vi "dfd_Convert ZPK String to Filter.vi"(8 "error in (no error)":errorcluster, 10 "xml string in":string, 11 "filter":T1={"mSRate_Fs"=1.0, "mSRate_Version"="1.0", "mSRate_Comments"="", "mSRate_OrgCoef"={"type"=enum."Undefined", "gain"=1.0, "coef a (k)"=[], "coef b (v)"=[]}, "mSRate_CurCoef"={"type"=enum."Undefined", "gain"=1.0, "coef a (k)"=[], "coef b (v)"=[]}, "mSRate_Quantized?"=FALSE, "mSRate_QCoef"={"type"=enum."Undefined", "gain"=1.0, "coef a (k)"=[], "coef b (v)"=[]}, "mSRate_QSettings"=[], "mSRate_Order"=0, "mSRate_Scaling"={"mSRate_ScaleByPowerOf2?"=FALSE, "mSRate_ScaleType"=enum."No Norm"}} {"mSRate_QSettings"."source" items=["Coef a/k"=0, "Coef b/v"=7, "Input"=1, "Output"=2, "Multiplicand"=3, "Product"=4, "Sum"=5, "Delay"=6, "Gain"=8]}) -> (0 "error out":errorcluster, 3 "filter out":T1={"mSRate_Fs"=1.0, "mSRate_Version"="1.0", "mSRate_Comments"="", "mSRate_OrgCoef"={"type"=enum."Undefined", "gain"=1.0, "coef a (k)"=[], "coef b (v)"=[]}, "mSRate_CurCoef"={"type"=enum."Undefined", "gain"=1.0, "coef a (k)"=[], "coef b (v)"=[]}, "mSRate_Quantized?"=FALSE, "mSRate_QCoef"={"type"=enum."Undefined", "gain"=1.0, "coef a (k)"=[], "coef b (v)"=[]}, "mSRate_QSettings"=[], "mSRate_Order"=0, "mSRate_Scaling"={"mSRate_ScaleByPowerOf2?"=FALSE, "mSRate_ScaleType"=enum."No Norm"}} {"mSRate_QSettings"."source" items=["Coef a/k"=0, "Coef b/v"=7, "Input"=1, "Output"=2, "Multiplicand"=3, "Product"=4, "Sum"=5, "Delay"=6, "Gain"=8]})   [LabVIEW 2017, in "NI_DigFilter_Process.lvlib"]
uses:
  <vilib>/addons/Digital Filter Design/NI_DigFilter_Process.lvlib
  <vilib>/addons/Digital Filter Design/_Objects.llb/DFD Filter Obj.ctl
  <vilib>/addons/Digital Filter Design/_Objects.llb/DFD Filter Coef.ctl
  <vilib>/addons/Digital Filter Design/_Objects.llb/DFD Filter Structure Type Selector.ctl
  <vilib>/addons/Digital Filter Design/_Objects.llb/dfd_Internal Quantization Settings.ctl
  <vilib>/addons/Digital Filter Design/_Objects.llb/dfd_Internal Quantization Srcs.ctl
  <vilib>/addons/Digital Filter Design/_Objects.llb/DFD Coef Norm Type.ctl
  <vilib>/addons/Digital Filter Design/NI_DigFilterLicensed.lvlib
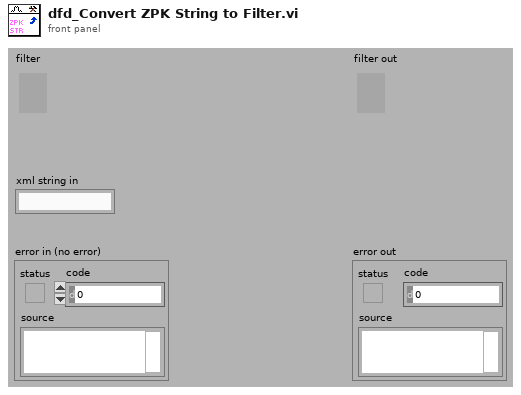
[diagram p1: front panel]
types:
  T1 = typedef "NI_DigFilterLicensed.lvlib/DFD Filter Obj.ctl" = cluster{"mSRate_Fs":dbl, "mSRate_Version":string, "mSRate_Comments":string, "mSRate_OrgCoef":T2, "mSRate_CurCoef":T2, "mSRate_Quantized?":bool, "mSRate_QCoef":T2, "mSRate_QSettings":T4[], "mSRate_Order":i32, "mSRate_Scaling":cluster{"mSRate_ScaleByPowerOf2?":bool, "mSRate_ScaleType":T6}}
  T2 = typedef "NI_DigFilterLicensed.lvlib/DFD Filter Coef.ctl" = cluster{"type":T3, "gain":dbl, "coef a (k)":dbl[], "coef b (v)":dbl[]}
  T3 = typedef "NI_DigFilterLicensed.lvlib/DFD Filter Structure Type Selector.ctl" = enum16{"Undefined", "FIR Direct Form", "FIR Direct Form Transposed", "FIR Symmetric", "FIR Antisymmetric", "IIR Direct Form I", "IIR Direct Form I Transposed", "IIR Direct Form II", "IIR Direct Form II Transposed", "IIR Cascaded Second Order Sections Form I", "IIR Cascaded Second Order Sections Form I Transposed", "IIR Cascaded Second Order Sections Form II", "IIR Cascaded Second Order Sections Form II Transposed", "Lattice Allpass (basic sections)", "Lattice Allpass (one multiplier sections)", "Lattice Allpass (normalized sections)", "Lattice AR (basic sections)", "Lattice AR (one multiplier sections)", "Lattice AR (normalized sections)", "Lattice MA (minimum phase)", "Lattice MA (maximum phase)", "Lattice ARMA (basic sections)", "Lattice ARMA (one multiplier sections)", "Lattice ARMA (normalized sections)"}
  T4 = typedef "NI_DigFilterLicensed.lvlib/dfd_Internal Quantization Settings.ctl" = cluster{"source":T5, "wl":i16, "iwl":i16, "overflow mode":enum16{"Saturation", "Wrap"}, "rounding mode":enum16{"Nearest", "Truncation"}, "signed?":bool}
  T5 = typedef "NI_DigFilterLicensed.lvlib/dfd_Internal Quantization Srcs.ctl" = u16
  T6 = typedef "NI_DigFilterLicensed.lvlib/DFD Coef Norm Type.ctl" = enum16{"No Norm", "Time Domain 1-Norm", "Time Domain 2-Norm", "Time Domain Inf-Norm"}
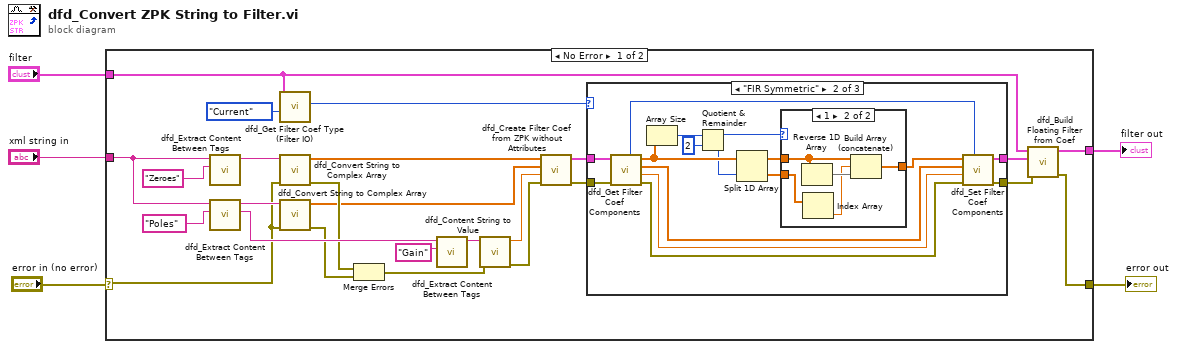
[diagram p0: block diagram]
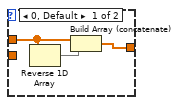
[diagram p3: hidden frame]
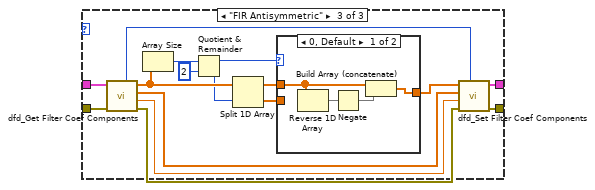
[diagram p4: hidden frame]
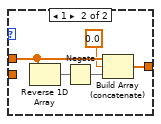
[diagram p5: hidden frame]
diagram:
  n1 = case shown="No Error" "error in (no error)" {
    selector: "error in (no error)" -> [w16 w82]
    tunnel: "xml string in" -> [w30 _]
    tunnel: [w18 _] -> w4
    tunnel: "filter" -> [w14 _]
    tunnel: [w19 w82] -> w2
    frame No Error {
      n2 = call <vilib>:"dfd_Extract Content Between Tags.vi"("element"="Zeroes", "xml string with tag"=w30) -> ("content"=w24:string)  [unwired: 9 out]
      n3 = call <vilib>:"dfd_Extract Content Between Tags.vi"("element"="Poles", "xml string with tag"=w30) -> ("remaining string"=w29:string, "content"=w23:string)  [unwired: 8 out]
      n4 = call <vilib>:"dfd_Get Filter Coef Type (Filter IO).vi"("coef source"=enum16{"Original", "Current", "Quantized"}."Current", "filter in"=w14) -> ("type"=w8:T3)  [unwired: 1 in, 8 out]
      n5 = call <vilib>:"dfd_Convert String to Complex Array .vi"("error in"=w16, "string"=w24) -> ("error out"=w21:errorcluster, "roots"=w6:cdb[])  [unwired: 8 out]
      n6 = call <vilib>:"dfd_Convert String to Complex Array .vi"("error in"=w16, "string"=w23) -> ("error out"=w22:errorcluster, "roots"=w7:cdb[])  [unwired: 8 out]
      n7 = Merge Errors(w21, w22) -> (w15:errorcluster)
      n8 = call <vilib>:"dfd_Extract Content Between Tags.vi"("element"="Gain", "xml string with tag"=w29) -> ("content"=w28:string)  [unwired: 9 out]
      n9 = call <vilib>:"dfd_Content String to Value.vi"("error in (no error)"=w15, "string"=w28) -> ("error out"=w20:errorcluster, "value"=w17:dbl)  [unwired: 8 out]
      n10 = call <vilib>:"dfd_Create Filter Coef from ZPK without Attributes.vi"("error in (no error)"=w20, "gain"=w17, "poles"=w7, "zeros"=w6) -> ("error out"=w11:errorcluster, "filter coef out"=w12:T2)  [unwired: 6 out]
      n11 = case shown="\"FIR Symmetric\"" w8 {
        tunnel: w12 -> [w31 w48 w72]
        tunnel: w11 -> [w32 w47 w71]
        tunnel: [w32 w33 w57] -> w10
        tunnel: [w31 w34 w58] -> w9
        frame "Undefined", Default {
        }
        frame "FIR Symmetric" {
          n12 = call <vilib>:"dfd_Get Filter Coef Components.vi"("error in (no error)"=w47, "filter coef"=w48) -> ("error out"=w35:errorcluster, "gain"=w36:dbl, "coef a (k)"=w37:dbl[], "coef b (v)"=w43:dbl[], "type"=w38:T3)  [unwired: 5 out]
          n13 = Array Size(array=w43) -> (size(s)=w46:i32)
          n14 = Quotient & Remainder(x=w46, y=2) -> (x-y*floor(x/y)=w44:i32, floor(x/y)=w42:i32)
          n15 = Split 1D Array(array=w43, index=w42) -> (first subarray=w41:dbl[], second subarray=w40:dbl[])
          n16 = case shown="1" w44 {
            tunnel: w41 -> [w51 w56]
            tunnel: w40 -> [_ w54]
            tunnel: [w49 w55] -> w39
            frame 0, Default {
              n17 = Reverse 1D Array(array=w51) -> (reversed array=w50:dbl[])
              n18 = Build Array (concatenate)(w51, w50) -> (w49:dbl[])
            }
            frame 1 {
              n19 = Reverse 1D Array(array=w56) -> (reversed array=w53:dbl[])
              n20 = Index Array(array=w54) -> (element=w52:dbl)  [unwired: 1 in]
              n21 = Build Array (concatenate)(w56, w52, w53) -> (w55:dbl[])
            }
          }
          n22 = call <vilib>:"dfd_Set Filter Coef Components.vi"("type"=w38, "error in (no error)"=w35, "gain"=w36, "coef a (k)"=w37, "coef b (v)"=w39) -> ("error out"=w33:errorcluster, "filter coef"=w34:T2)  [unwired: 5 out]
        }
        frame "FIR Antisymmetric" {
          n23 = call <vilib>:"dfd_Get Filter Coef Components.vi"("error in (no error)"=w71, "filter coef"=w72) -> ("error out"=w59:errorcluster, "gain"=w60:dbl, "coef a (k)"=w61:dbl[], "coef b (v)"=w67:dbl[], "type"=w62:T3)  [unwired: 5 out]
          n24 = Array Size(array=w67) -> (size(s)=w70:i32)
          n25 = Quotient & Remainder(x=w70, y=2) -> (x-y*floor(x/y)=w68:i32, floor(x/y)=w66:i32)
          n26 = Split 1D Array(array=w67, index=w66) -> (first subarray=w65:dbl[], second subarray=w64:dbl[])
          n27 = case shown="0, Default" w68 {
            tunnel: w65 -> [w76 w81]
            tunnel: w64 -> [_ _]
            tunnel: [w74 w80] -> w63
            frame 0, Default {
              n28 = Reverse 1D Array(array=w76) -> (reversed array=w75:dbl[])
              n29 = Negate(x=w75) -> (-x=w73:dbl[])
              n30 = Build Array (concatenate)(w76, w73) -> (w74:dbl[])
            }
            frame 1 {
              n31 = Reverse 1D Array(array=w81) -> (reversed array=w79:dbl[])
              n32 = Negate(x=w79) -> (-x=w77:dbl[])
              n33 = Build Array (concatenate)(w81, 0.0, w77) -> (w80:dbl[])
            }
          }
          n34 = call <vilib>:"dfd_Set Filter Coef Components.vi"("type"=w62, "error in (no error)"=w59, "gain"=w60, "coef a (k)"=w61, "coef b (v)"=w63) -> ("error out"=w57:errorcluster, "filter coef"=w58:T2)  [unwired: 5 out]
        }
      }
      n35 = call <vilib>:"dfd_Build Floating Filter from Coef.vi"("error in (no error)"=w10, "filter coef"=w9, "filter in"=w14) -> ("error out"=w19:errorcluster, "filter out"=w18:T1)  [unwired: 1 in, 6 out]
    }
    frame Error {
    }
  }
  "filter out" <- w4
  "error out" <- w2
